vi "ProjectSelectInterface.vi"(8 "error in (no error)":errorcluster, 11 "Project.lvclass In":refnum<class "Project.lvclass">) -> (0 "error out":errorcluster, 2 "DeployProject":string, 3 "Project.lvclass Out":refnum<class "Project.lvclass">)   [LabVIEW 2014, in "Project.lvclass"]
uses:
  Project.lvclass
panel:
  in  "Run":bool
  in  "ProjectList":i32(listbox)
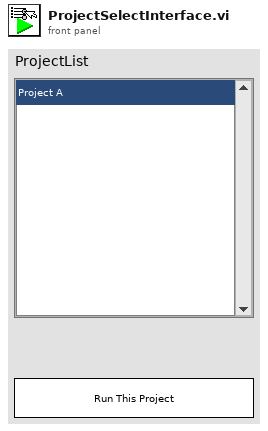
[diagram p1: front panel]
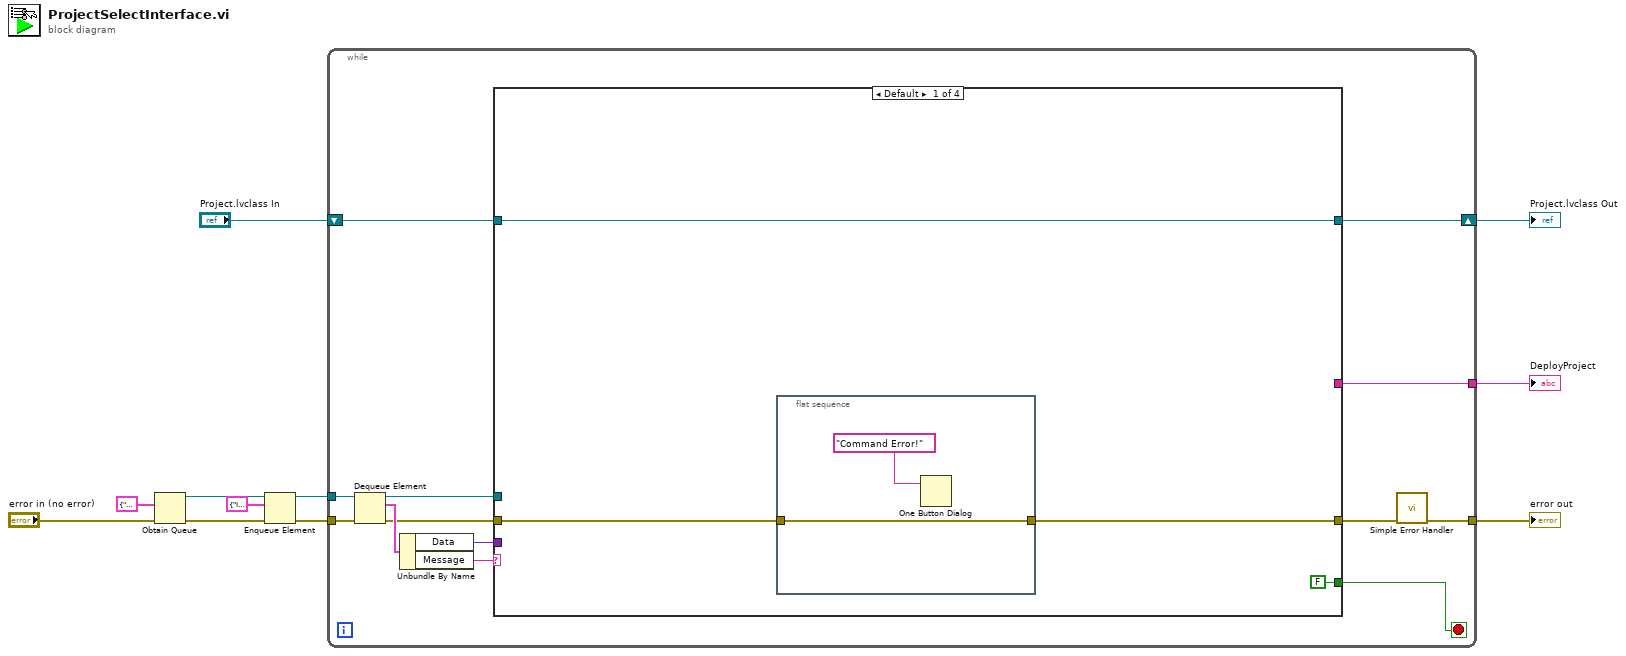
[diagram p0: block diagram]
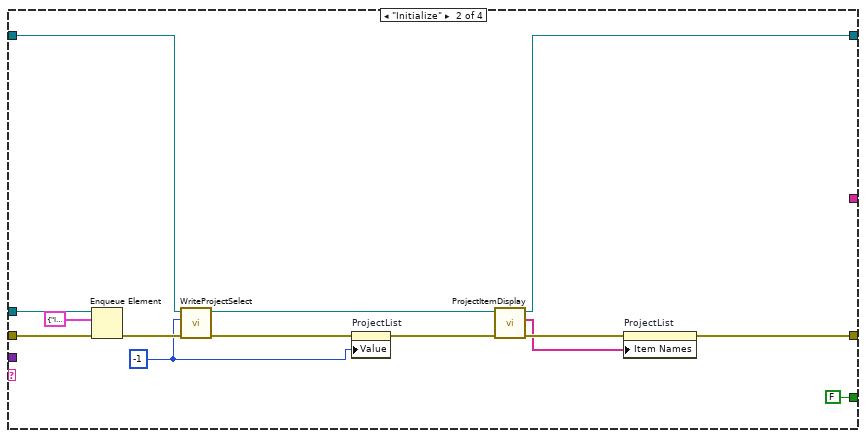
[diagram p2: hidden frame]
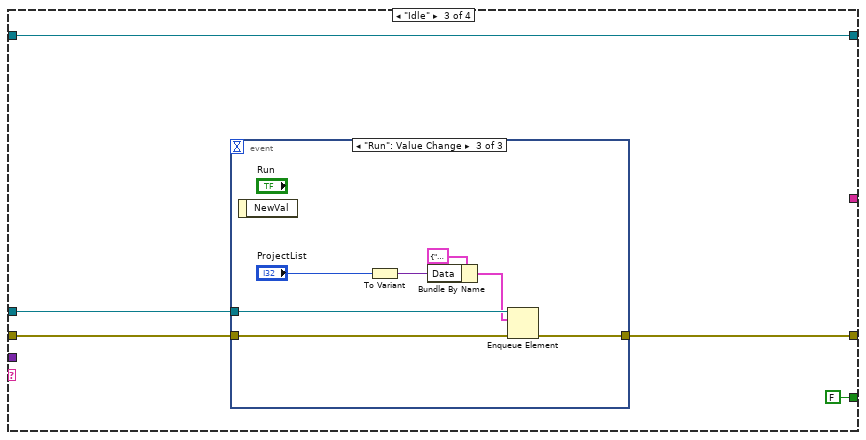
[diagram p3: hidden frame]
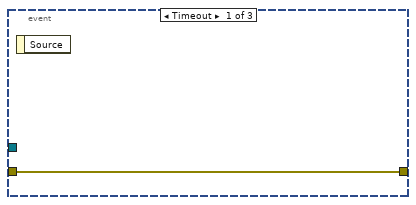
[diagram p4: hidden frame]
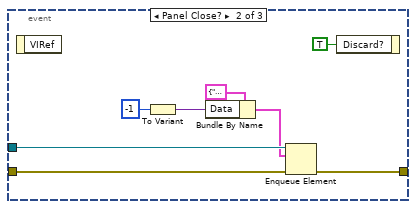
[diagram p5: hidden frame]
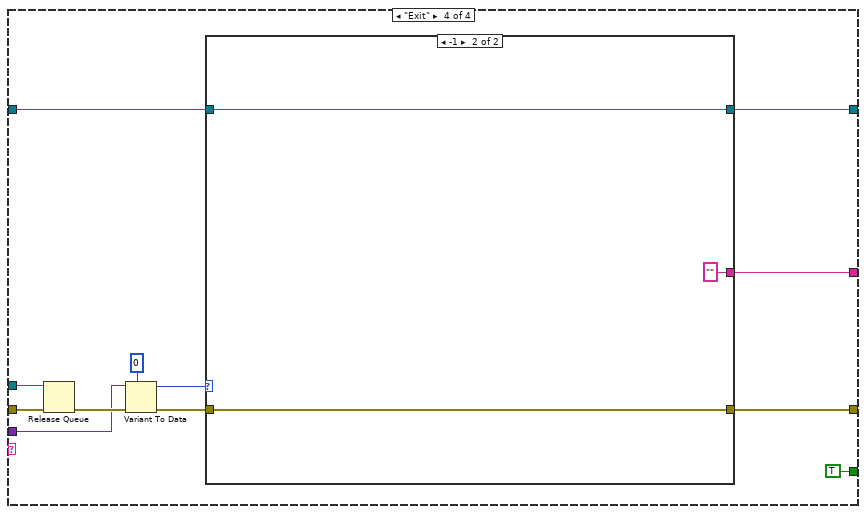
[diagram p6: hidden frame]
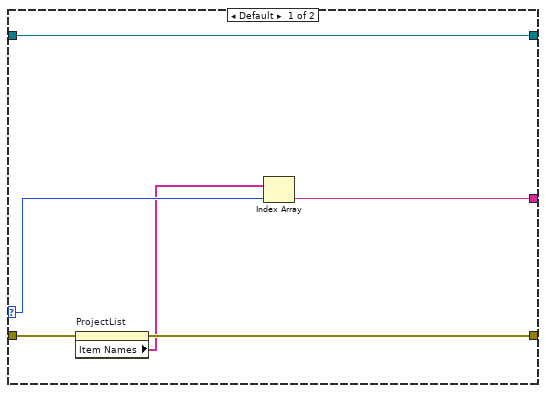
[diagram p7: hidden frame]
diagram:
  n1 = Obtain Queue(element data type=cluster{"Message":string, "Data":variant} {"Message"="", "Data"=variant}, error in (no error)="error in (no error)") -> (queue out=w10:refnum<queue>, error out=w11:errorcluster)  [unwired: 3 in, 1 out]
  n2 = Enqueue Element(queue=w10, element=cluster{"Message":string, "Data":variant} {"Message"="Initialize", "Data"=variant}, error in (no error)=w11) -> (queue out=w7:refnum<queue>, error out=w6:errorcluster)  [unwired: 1 in, 1 out]
  n3 = while {
    tunnel: w7 -> [w24]
    tunnel: w6 -> [w23]
    tunnel: [w15] -> w5
    shift-right: [w12] -> w1
    shift-left: "Project.lvclass In" -> [w13]
    tunnel: [w14] -> w2
    stop <- w17 stop-if-true
    n4 = Dequeue Element(queue=w24, error in (no error)=w23) -> (queue out=w18:refnum<queue>, element=w22:cluster{"Message":string, "Data":variant}, error out=w20:errorcluster)  [unwired: 1 in, 1 out]
    n5 = Unbundle By Name(w22) -> ("Data"=w16:variant, "Message"=w21:string)
    n6 = case shown="Default" w21 {
      tunnel: w20 -> [w28 w44 w48 w76]
      tunnel: [w27 w33 w47 w69] -> w19
      tunnel: w18 -> [_ w43 w49 w75]
      tunnel: [FALSE FALSE FALSE TRUE] -> w17
      tunnel: w16 -> [_ _ _ w73]
      tunnel: [_ _ _ w68] -> w15
      tunnel: w13 -> [w25 w39 w45 w67]
      tunnel: [w25 w31 w45 w66] -> w12
      frame Default {
        n7 = flat-sequence {
          tunnel: w28 -> [w30]
          tunnel: [w30] -> w27
          frame #0 {
            n8 = One Button Dialog(message="Command Error!") -> ()  [unwired: 1 in, 1 out]
          }
        }
      }
      frame "Initialize" {
        w35 = -1 ("ProjectSelectIdx")
        n9 = Enqueue Element(queue=w43, element=cluster{"Message":string, "Data":variant} {"Message"="Idle", "Data"=variant}, error in (no error)=w44) -> (error out=w40:errorcluster)  [unwired: 1 in, 2 out]
        n10 = call "WriteProjectSelect.vi"("error in (no error)"=w40, "ProjectSelectIdx"=w35, "Project.lvclass In"=w39) -> ("error out"=w38:errorcluster, "Project.lvclass Out"=w37:refnum<class "Project.lvclass">)  [unwired: 7 in]
        n11 = property on="ProjectList" class="LstBox (strict)"(error in=w38, "Value"=w35) -> (error out=w36:errorcluster)  [unwired: 1 in, 1 out]
        n12 = call "ProjectItemDisplay.vi"("error in (no error)"=w36, "Project.lvclass In"=w37) -> ("error out"=w34:errorcluster, "ProjectNames"=w32:string[], "Project.lvclass Out"=w31:refnum<class "Project.lvclass">)  [unwired: 5 in, 2 out]
        n13 = property on="ProjectList" class="LstBox (strict)"(error in=w34, "Item Names"=w32) -> (error out=w33:errorcluster)  [unwired: 1 in, 1 out]
      }
      frame "Idle" {
        n14 = event shown="[2] \"Run\": Value Change" {
          selector: _ -> [_ _ _]
          dyn-events: _ -> [_ _ _]
          timeout: _ -> [_ _ _]
          tunnel: w49 -> [_ w55 w63]
          tunnel: w48 -> [w50 w57 w65]
          tunnel: [w50 w56 w64] -> w47
          event Timeout {
            n15 = event-data() -> ()  [unwired: 1 in, 1 out]
          }
          event Panel Close? {
            n16 = event-data() -> ()  [unwired: 1 in, 1 out]
            n17 = To Variant(anything=-1) -> (Variant=w52:variant)
            n18 = Bundle By Name(cluster=cluster{"Message":string, "Data":variant} {"Message"="Exit", "Data"=variant} ("element"), "Data"=w52) -> (w51:cluster{"Message":string, "Data":variant})
            n19 = Enqueue Element(queue=w55, element=w51, error in (no error)=w57) -> (error out=w56:errorcluster)  [unwired: 1 in, 2 out]
            n20 = event-data("Discard?"=TRUE) -> ()  [unwired: 1 in, 1 out]
          }
          event "Run": Value Change {
            n21 = event-data() -> ()  [unwired: 1 in, 1 out]
            n22 = To Variant(anything="ProjectList") -> (Variant=w60:variant)
            n23 = Bundle By Name(cluster=cluster{"Message":string, "Data":variant} {"Message"="Exit", "Data"=variant} ("element"), "Data"=w60) -> (w61:cluster{"Message":string, "Data":variant})
            n24 = Enqueue Element(queue=w63, element=w61, error in (no error)=w65) -> (error out=w64:errorcluster)  [unwired: 1 in, 2 out]
          }
        }
      }
      frame "Exit" {
        n25 = Release Queue(queue=w75, error in (no error)=w76) -> (error out=w74:errorcluster)  [unwired: 1 in, 2 out]
        n26 = Variant To Data(error in=w74, type=0, Variant=w73) -> (data=w70:i32, error out=w71:errorcluster)
        n27 = case shown="-1" w70 {
          selector: w70 -> [w81 _]
          tunnel: w71 -> [w83 w86]
          tunnel: [w82 w86] -> w69
          tunnel: [w79 ""] -> w68
          tunnel: w67 -> [w78 w84]
          tunnel: [w78 w84] -> w66
          frame Default {
            n28 = property on="ProjectList" class="LstBox (strict)"(error in=w83) -> (error out=w82:errorcluster, "Item Names"=w80:string[])  [unwired: 1 in, 1 out]
            n29 = Index Array(array=w80, index=w81) -> (element=w79:string)
          }
          frame -1 {
          }
        }
      }
    }
    n30 = call <vilib>:"Simple Error Handler.vi"("error in (no error)"=w19) -> ("error out"=w14:errorcluster)  [unwired: 4 in, 4 out]
  }
  "DeployProject" <- w5
  "Project.lvclass Out" <- w1
  "error out" <- w2
